vi "SeimensS7Net_Create.vi"(5 "Slot":u8=1, 7 "Rack":u8, 8 "error in (no error)":errorcluster caption="错误输入（无错误）", 9 "ipAddress":string="192.168.6.100", 10 "siemens":i32(ring)=1 items=["S1200"=1, "S300"=2, "S400"=3, "S1500"=4, "S200Smart"=5, "S200"=6], 11 "Seimens 输入":refnum<class "Seimens.lvclass">) -> (0 "error out":errorcluster caption="错误输出", 3 "Seimens 输出":refnum<class "Seimens.lvclass">)   [LabVIEW 2018, in "Seimens.lvclass"]
uses:
  Seimens.lvclass
  D:/LiMing/Labview/lib/LM_HslCommunication/DLL/HslCommunication.dll
  DLL/HslCommunication.dll
  Seimens.lvclass/Seimens.ctl
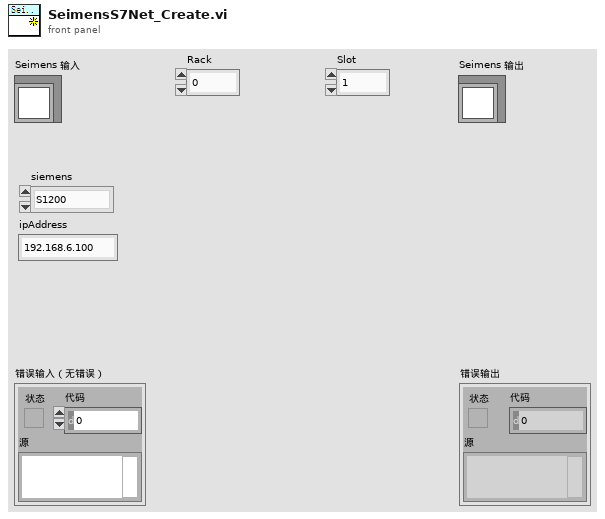
[diagram p1: front panel]
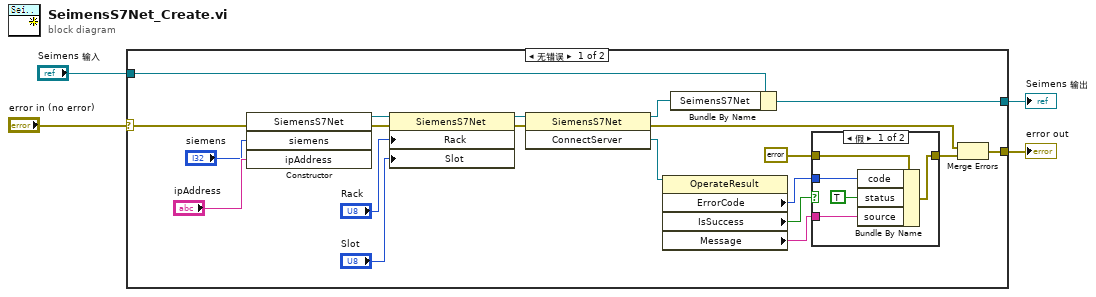
[diagram p0: block diagram]
diagram:
  n1 = case shown="无错误" "error in (no error)" {
    selector: "error in (no error)" -> [w13 w32]
    tunnel: [w10 w32] -> w3
    tunnel: [w5 w31] -> w1
    tunnel: "Seimens 输入" -> [w12 w31]
    frame No Error {
      n2 = constructor class="SiemensS7Net"(error in=w13, "siemens"="siemens", "ipAddress"="ipAddress") -> (reference out=w17:refnum<k24>, error out=w18:errorcluster)  [unwired: 2 in, 3 out]
      n3 = property class="SiemensS7Net"(reference=w17, error in=w18, "Rack"="Rack", "Slot"="Slot") -> (reference out=w19:refnum<k24>, error out=w21:errorcluster)
      n4 = invoke class="SiemensS7Net" method="ConnectServer"(reference=w19, error in=w21) -> (reference out=w11:refnum<k24>, error out=w23:errorcluster, "ConnectServer"=w20:refnum<k24>)  [unwired: 1 in]
      n5 = property class="OperateResult"(reference=w20) -> ("ErrorCode"=w8:i32, "IsSuccess"=w6:bool, "Message"=w7:string)  [unwired: 1 in, 2 out]
      n6 = Bundle By Name(cluster=w12, "SeimensS7Net"=w11) -> (w5:refnum<class "Seimens.lvclass">)
      n7 = case shown="假" w6 {
        tunnel: [w29 w30] -> w24
        tunnel: errorcluster {"status"=FALSE, "code"=0, "source"=""} ("错误输出") -> [w28 w30]
        tunnel: w8 -> [w27 _]
        tunnel: w7 -> [w26 _]
        frame False {
          n8 = Bundle By Name(cluster=w28, "code"=w27, "status"=TRUE, "source"=w26) -> (w29:errorcluster)
        }
        frame True {
        }
      }
      n9 = Merge Errors(w23, w24) -> (w10:errorcluster)
    }
    frame Error {
    }
  }
  "error out" <- w3
  "Seimens 输出" <- w1
